vi "TDMS Find Property.vi"(4 "Property Name":string, 6 "Property Names":string[](array[string]), 7 "Property Values":variant[](array[variant])) -> (1 "Index":i32, 2 "Property Value":variant)   [LabVIEW 2011]
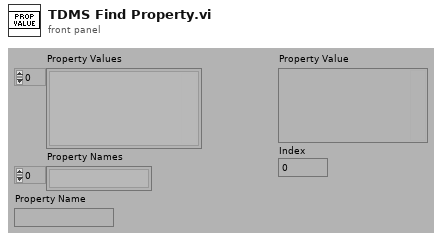
[diagram p1: front panel]
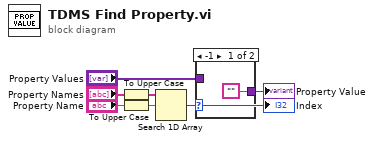
[diagram p0: block diagram]
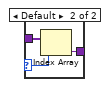
[diagram p2: hidden frame]
diagram:
  n1 = To Upper Case(1:"Property Names") -> (0:w3:string[])
  n2 = To Upper Case(1:"Property Name") -> (0:w1:string)
  n3 = Search 1D Array(1D array=w3, element=w1) -> (index of element=w5:i32)  [unwired: 1 out]
  "Index" <- w5
  n4 = case shown="-1" w5 {
    selector: w5 -> [_ w9]
    tunnel: "Property Values" -> [_ w11]
    tunnel: ["" w10] -> w6
    frame -1 {
    }
    frame Default {
      n5 = Index Array(array=w11, index=w9) -> (element=w10:variant)
    }
  }
  "Property Value" <- w6
